vi "新设备提示.vi"() -> ()   [LabVIEW 2013]
panel:
  out "管-监测模式状态":refnum<vi>
  in  "确定":bool
  # "* 通知：待命名新设备上线"
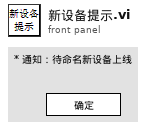
[diagram p1: front panel]
types:
  T1 = enum32{"Invalid", "Standard", "Closed", "Hidden", "Minimized", "Maximized"}
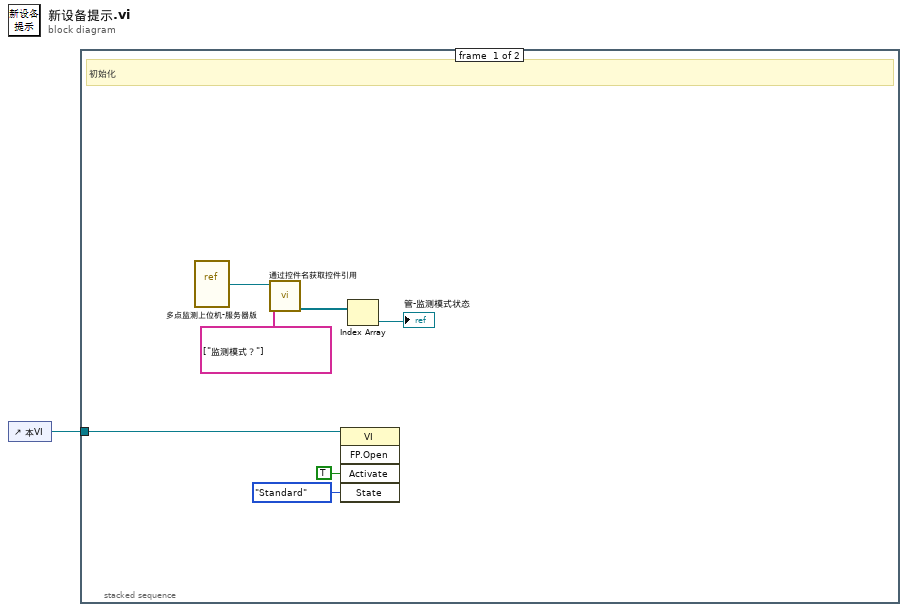
[diagram p0: block diagram]
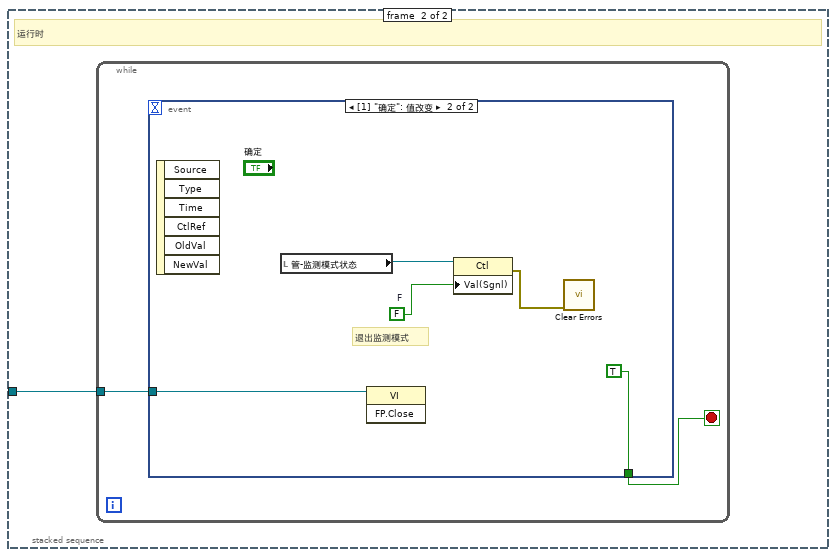
[diagram p2: hidden frame]
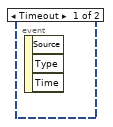
[diagram p3: hidden frame]
diagram:
  n1 = control-ref of="本VI"() -> (w1:refnum<vi>)
  n2 = stacked-sequence {
    tunnel: w1 -> [w5 w9]
    frame #0 {
      # "初始化"
      n3 = vi-ref "多点监测上位机-服务器版.vi"() -> (w8:refnum<vi>)
      n4 = call "通过控件名获取控件引用.vi"("控件名数组"=string[] ["监测模式？"], "VI引用"=w8) -> ("控件引用输出"=w6:refnum<vi>[])  [unwired: 7 in, 2 out]
      n5 = invoke class="VI" method="FP.Open"(reference=w5, "Activate"=TRUE ("激活？"), "State"=T1."Standard" ("状态")) -> ()  [unwired: 2 in, 5 out]
      n6 = Index Array(array=w6) -> (element=→"管-监测模式状态":refnum<vi>)  [unwired: 1 in]
    }
    frame #1 {
      # "运行时"
      n7 = while {
        tunnel: w9 -> [w10]
        stop <- w11 stop-if-true
        n8 = event shown="[1] \"确定\": 值改变" {
          selector: _ -> [_ _]
          dyn-events: _ -> [_ _]
          timeout: _ -> [_ _]
          tunnel: [_ TRUE ("确定")] -> w11
          tunnel: w10 -> [_ w15]
          event Timeout {
            n9 = event-data() -> ()  [unwired: 1 in, 3 out]
          }
          event "确定": Value Change {
            w13 = FALSE  # F
            # "退出监测模式"
            n10 = event-data() -> ()  [unwired: 1 in, 6 out]
            n11 = local read "管-监测模式状态"() -> (w14:refnum<vi>)
            n12 = invoke class="VI" method="FP.Close"(reference=w15) -> ()  [unwired: 2 in, 3 out]
            n13 = property class="Ctl"(reference=w14, "Val(Sgnl)"=w13) -> (error out=w12:errorcluster)  [unwired: 1 in, 1 out]
            n14 = call <vilib>:"Clear Errors.vi"("error in (no error)"=w12) -> ()  [unwired: 6 in, 1 out]
          }
        }
      }
    }
  }
